vi "Add Button State.vi"(8 "error in (no error)":errorcluster, 10 "State":refnum<class "BitMap.lvclass">, 11 "Control in":refnum<class "Control.lvclass">) -> (0 "error out":errorcluster, 3 "Control out":refnum<class "Control.lvclass">)   [LabVIEW 2013, in "uitools_Control.lvlib" / "Control.lvclass"]
uses:
  Control.lvclass
  <userlib>/BitMan/BitMap class/BitMap.lvclass
  Control.lvclass/Control.ctl
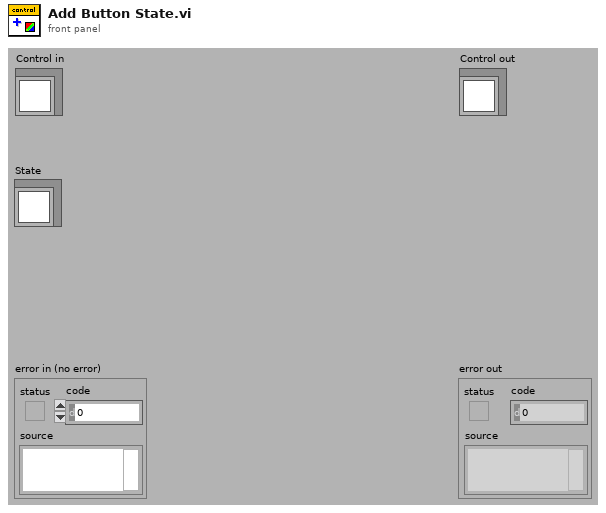
[diagram p1: front panel]
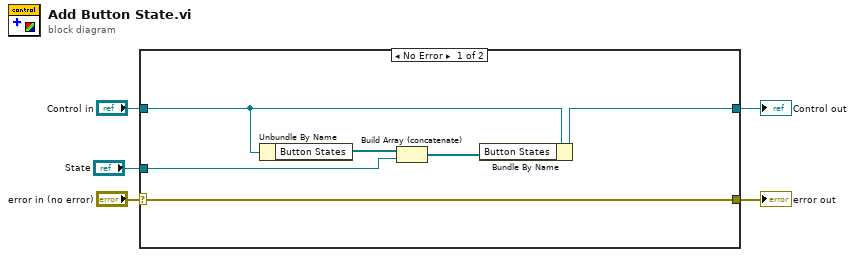
[diagram p0: block diagram]
diagram:
  n1 = case shown="No Error" "error in (no error)" {
    selector: "error in (no error)" -> [w11 w13]
    tunnel: [w11 w13] -> w4
    tunnel: [w7 w12] -> w2
    tunnel: "Control in" -> [w10 w12]
    tunnel: "State" -> [w6 _]
    frame No Error {
      n2 = Unbundle By Name(w10) -> ("Button States"=w9:refnum<class "BitMap.lvclass">[])
      n3 = Build Array (concatenate)(w9, w6) -> (w8:refnum<class "BitMap.lvclass">[])
      n4 = Bundle By Name(cluster=w10, "Button States"=w8) -> (w7:refnum<class "Control.lvclass">)
    }
    frame Error {
    }
  }
  "error out" <- w4
  "Control out" <- w2
